vi "4Pi Obj Lock - Setup Camera.vi"(0 "Camera Notifier Name":string, 2 "Save ROI?":bool) -> (8 "Canceled?":bool)   [LabVIEW 2016]
uses:
  <vilib>/Utility/miscctls.llb/LVPointTypeDef.ctl
  Device Library/Cameras/Camera Controls/Generic Camera ROI.ctl
  Device Library/Cameras/Camera Controls/Generic Camera Actions.ctl
  4Pi Objective Lock Type Defs/4Pi Obj Lock - Camera Settings.ctl
panel:
  in  "Exposure Time (ms)":dbl
  in  "Tool Selection":enum32{"Zoom Tool", "ROI Tool", "Pan Tool"}(radio)
  in  "Cancel":bool
  in  "Done":bool
  out "Camera Display":T1(plugin-control)
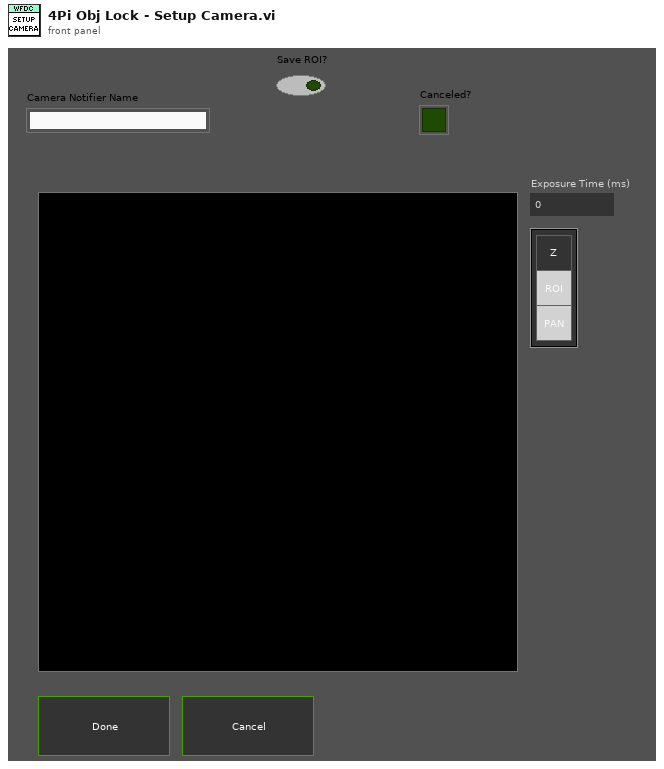
[diagram p1: front panel]
types:
  T1 = typedef "IMAQ Image.ctl" = refnum<image>
  T2 = typedef "Generic Camera Actions.ctl" = enum16{"Status", "Live Preview", "Capture", "Abort", "Set Exposure Time (s)", "Get Exposure Time (s)", "Record Settings", "Set ROI", "Get ROI", "Defect Correction On/Off", "Cooler On/Off", "Fan On/Off", "Quti"}
  T3 = typedef "Generic Camera ROI.ctl" = cluster{"H Offset":u16, "V Offset":u16, "H Width":u16, "V Width":u16}
  T4 = enum16{"Always On", "Always Off", "Off While Running"}
  T5 = typedef "LVPointTypeDef.ctl" = cluster{"Horizontal":i16, "Vertical":i16}
  T6 = typedef "LVRectTypeDef.ctl" = cluster{"Left":i16, "Top":i16, "Right":i16, "Bottom":i16}
  T7 = typedef "LVBoundsTypeDef.ctl" = cluster{"Width":u32, "Height":u32}
  T8 = typedef "4Pi Obj Lock - Camera Settings.ctl" = cluster{"Exposure Time (s)":dbl, "H Offset":u16, "V Offset":u16, "H Width":u16, "V Width":u16}
  T9 = cluster{"Global Rectangle":i32[], "Contours":cluster{"Contour Type":u32, "ROI Type":u32, "Points":i32[]}[]}
  T10 = cluster{"Contour Type":u32, "ROI Type":u32, "Points":i32[]}[]
  T11 = cluster{"Contour Type":u32, "ROI Type":u32, "Points":i32[]}
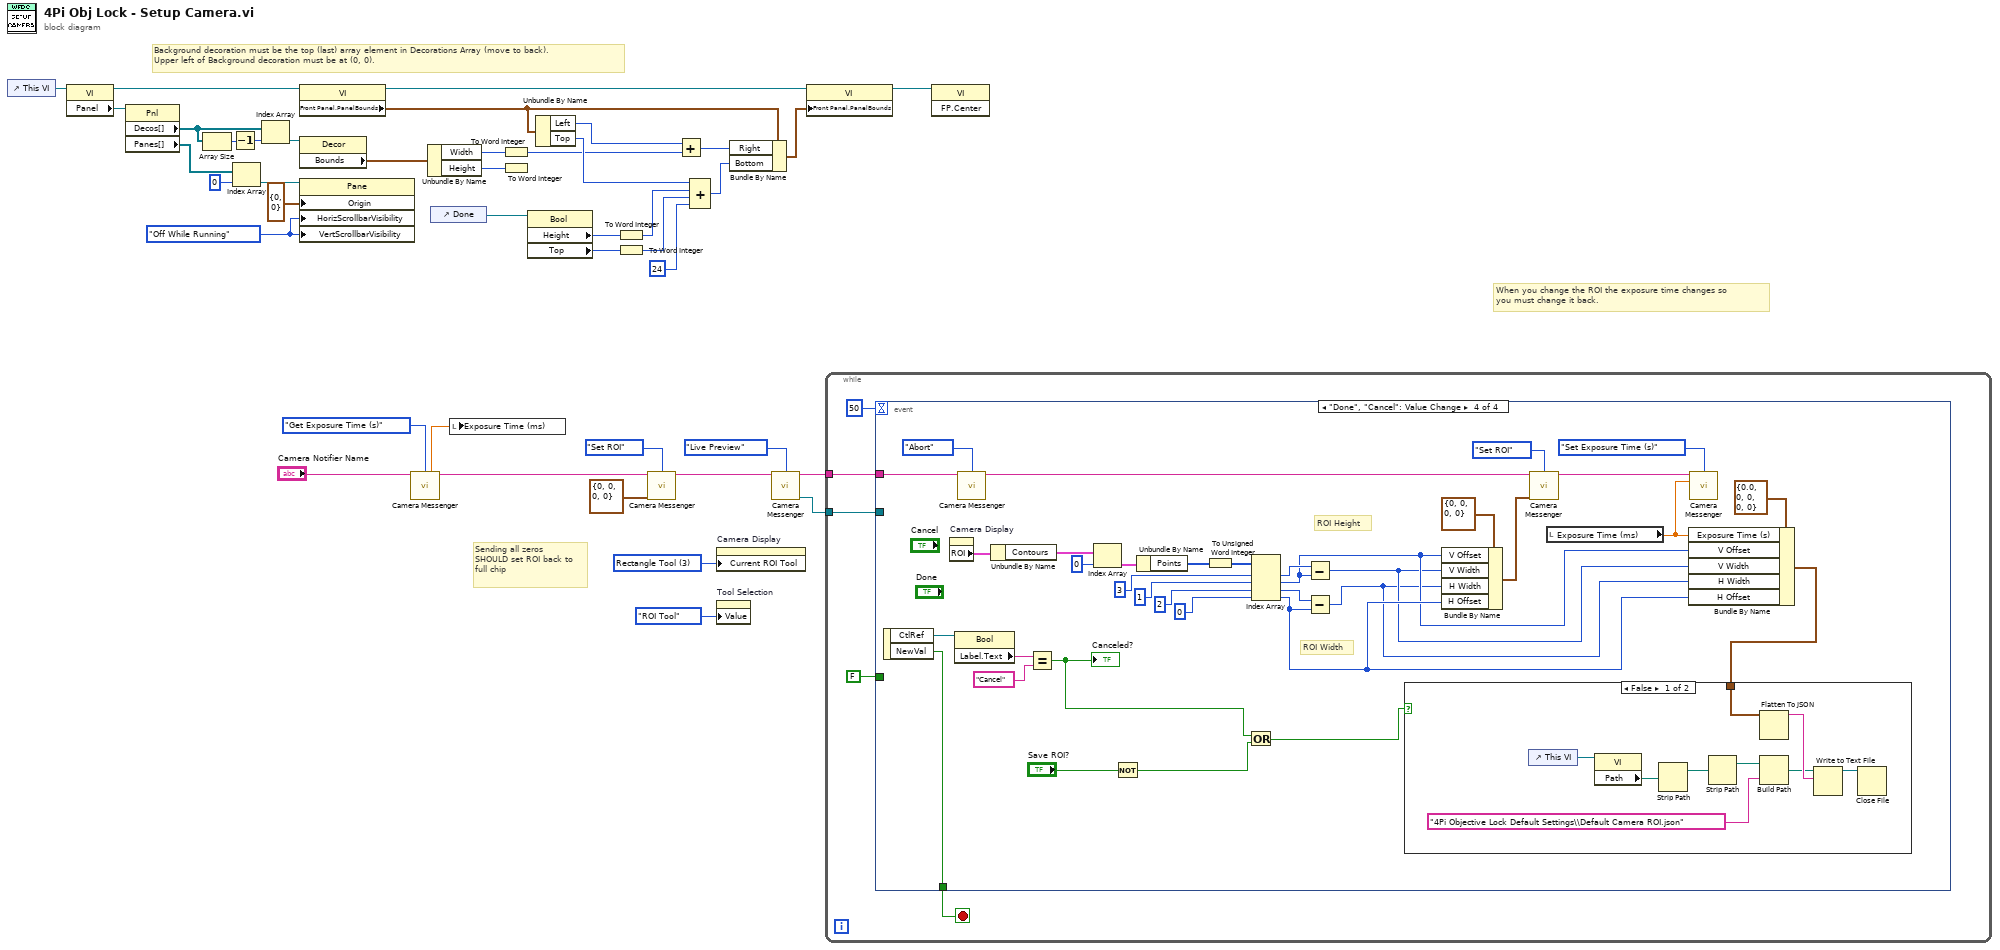
[diagram p0: block diagram]
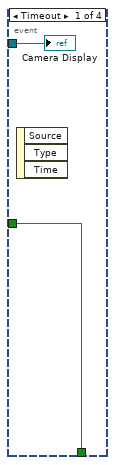
[diagram p2: hidden frame]
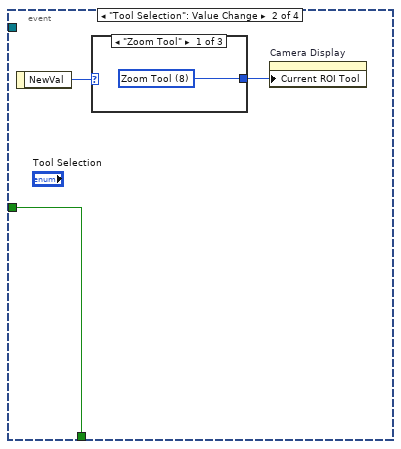
[diagram p3: hidden frame]
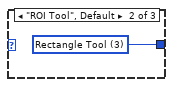
[diagram p4: hidden frame]
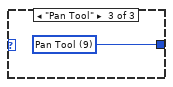
[diagram p5: hidden frame]
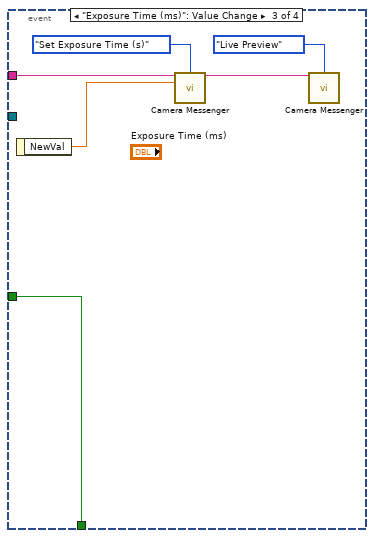
[diagram p6: hidden frame]
diagram:
  w23 = T4."Off While Running" ("Vertical Scrollbar Visibility")
  w42 = u32 3 items=["Zoom Tool"=8, "Selection Tool"=0, "Pan Tool"=9, "Point Tool"=1, "Line Tool"=2, "Rectangle Tool"=3, "Rotated Rectangle Tool"=12, "Polyline Tool"=10, "Polygon Tool"=5, "Freehand Tool"=11, "Closed Freehand Tool"=6, "Ellipse Tool"=4, "Annulus Tool"=7] ("Current ROI Tool")
  # "Background decoration must be the top (last) array element in Decorations Array (move to back).\nUpper left of Background decoration must be at (0, 0)."
  # "When you change the ROI the exposure time changes so\nyou must change it back."
  # "Sending all zeros SHOULD set ROI back to full chip"
  n1 = control-ref of="This VI"() -> (w15:refnum<vi>)
  n2 = property class="VI"(reference=w15) -> (reference out=w24:refnum<vi>, "Panel"=w16:refnum<vi>)  [unwired: 1 in, 1 out]
  n3 = property class="Pnl"(reference=w16) -> ("Decos[]"=w14:refnum<vi>[], "Panes[]"=w20:refnum<vi>[])  [unwired: 1 in, 2 out]
  n4 = Array Size(array=w14) -> (size(s)=w12:i32)
  n5 = Decrement(x=w12) -> (x-1=w13:i32)
  n6 = Index Array(array=w20, index=0) -> (element=w19:refnum<vi>)
  n7 = Index Array(array=w14, index=w13) -> (element=w22:refnum<vi>)
  n8 = property class="VI"(reference=w24) -> (reference out=w26:refnum<vi>, "Front Panel.PanelBounds"=w27:T6)  [unwired: 1 in, 1 out]
  n9 = property class="Decor"(reference=w22) -> ("Bounds"=w25:T7)  [unwired: 1 in, 2 out]
  n10 = property class="Pane"(reference=w19, "Origin"=T5 {"Horizontal"=0, "Vertical"=0}, "HorizScrollbarVisibility"=w23, "VertScrollbarVisibility"=w23) -> ()  [unwired: 1 in, 2 out]
  n11 = call "Camera Messenger.vi"("Notifier Name"="Camera Notifier Name", "General Camera Actions"=Generic_Camera_Actions."Get Exposure Time (s)") -> ("Current Exposure Time (s)"=w8:dbl, "Notifier Name Dup"=w7:string)  [unwired: 8 in, 4 out]
  n12 = Unbundle By Name(w25) -> ("Width"=w30:u32, "Height"=w33:u32)
  n13 = control-ref of="Done"() -> (w17:refnum<vi>)
  n14 = local write "Exposure Time (ms)"(w8) -> ()
  n15 = To Word Integer(number=w30) -> (16bit integer=w32:i16)
  n16 = To Word Integer(number=w33) -> ()  [unwired: 1 out]
  n17 = property class="Bool"(reference=w17) -> ("Height"=w35:u32, "Top"=w36:i32)  [unwired: 1 in, 2 out]
  n18 = Unbundle By Name(w27) -> ("Left"=w29:i16, "Top"=w40:i16)
  n19 = To Word Integer(number=w35) -> (16bit integer=w38:i16)
  n20 = To Word Integer(number=w36) -> (16bit integer=w39:i16)
  n21 = call "Camera Messenger.vi"("Notifier Name"=w7, "General Camera Actions"=Generic_Camera_Actions."Set ROI", "Camera ROI"=T3 {"H Offset"=0, "V Offset"=0, "H Width"=0, "V Width"=0} ("General Camera ROI")) -> ("Notifier Name Dup"=w4:string)  [unwired: 7 in, 5 out]
  n22 = Add(x=w29, y=w32) -> (x+y=w31:i16)
  n23 = Compound Arithmetic op=ADD(w40, w38, w39, i16 24 ("y")) -> (w34:i16)
  n24 = property on="Camera Display" class="ImageControl"("Current ROI Tool"=w42) -> ()  [unwired: 2 in, 2 out]
  n25 = property on="Tool Selection" class="RadioBtnsControl (strict)"("Value"=enum32{"Zoom Tool", "ROI Tool", "Pan Tool"}."ROI Tool" ("Tool Selection")) -> ()  [unwired: 2 in, 2 out]
  n26 = Bundle By Name(cluster=w27, "Right"=w31, "Bottom"=w34) -> (w28:T6)
  n27 = call "Camera Messenger.vi"("Notifier Name"=w4, "General Camera Actions"=Generic_Camera_Actions."Live Preview") -> ("Notifier Name Dup"=w3:string, "Image Ref"=w1:T1)  [unwired: 8 in, 4 out]
  n28 = property class="VI"(reference=w26, "Front Panel.PanelBounds"=w28) -> (reference out=w11:refnum<vi>)  [unwired: 1 in, 1 out]
  n29 = while {
    tunnel: w1 -> [w45]
    tunnel: w3 -> [w43]
    stop <- w47 stop-if-true
    n30 = event shown="[3] \"Done\", \"Cancel\": Value Change" {
      selector: _ -> [_ _ _ _]
      dyn-events: _ -> [_ _ _ _]
      timeout: 50 -> [_ _ _ _]
      tunnel: [w49 w52 w61 w93] -> w47
      tunnel: FALSE -> [w49 w52 w61 _]
      tunnel: w45 -> [w48 _ _ _]
      tunnel: w43 -> [_ _ w60 w81]
      event Timeout {
        n31 = event-data() -> ()  [unwired: 1 in, 3 out]
        "Camera Display" <- w48
      }
      event "Tool Selection": Value Change {
        n32 = event-data() -> ("NewVal"=w51:enum32{"Zoom Tool", "ROI Tool", "Pan Tool"})  [unwired: 1 in]
        n33 = case shown="\"Zoom Tool\"" w51 {
          tunnel: [w53 w54 w55] -> w50
          frame "Zoom Tool" {
            w53 = u32 8 items=["Zoom Tool"=8, "Selection Tool"=0, "Pan Tool"=9, "Point Tool"=1, "Line Tool"=2, "Rectangle Tool"=3, "Rotated Rectangle Tool"=12, "Polyline Tool"=10, "Polygon Tool"=5, "Freehand Tool"=11, "Closed Freehand Tool"=6, "Ellipse Tool"=4, "Annulus Tool"=7] ("Current ROI Tool")
          }
          frame "ROI Tool", Default {
            w54 = u32 3 items=["Zoom Tool"=8, "Selection Tool"=0, "Pan Tool"=9, "Point Tool"=1, "Line Tool"=2, "Rectangle Tool"=3, "Rotated Rectangle Tool"=12, "Polyline Tool"=10, "Polygon Tool"=5, "Freehand Tool"=11, "Closed Freehand Tool"=6, "Ellipse Tool"=4, "Annulus Tool"=7] ("Current ROI Tool")
          }
          frame "Pan Tool" {
            w55 = u32 9 items=["Zoom Tool"=8, "Selection Tool"=0, "Pan Tool"=9, "Point Tool"=1, "Line Tool"=2, "Rectangle Tool"=3, "Rotated Rectangle Tool"=12, "Polyline Tool"=10, "Polygon Tool"=5, "Freehand Tool"=11, "Closed Freehand Tool"=6, "Ellipse Tool"=4, "Annulus Tool"=7] ("Current ROI Tool")
          }
        }
        n34 = property on="Camera Display" class="ImageControl"("Current ROI Tool"=w50) -> ()  [unwired: 2 in, 2 out]
      }
      event "Exposure Time (ms)": Value Change {
        n35 = event-data() -> ("NewVal"=w58:dbl)  [unwired: 1 in]
        n36 = call "Camera Messenger.vi"("Notifier Name"=w60, "General Camera Actions"=Generic_Camera_Actions."Set Exposure Time (s)", "Exposure Time (s)"=w58) -> ("Notifier Name Dup"=w57:string)  [unwired: 7 in, 5 out]
        n37 = call "Camera Messenger.vi"("Notifier Name"=w57, "General Camera Actions"=Generic_Camera_Actions."Live Preview") -> ()  [unwired: 8 in, 6 out]
      }
      event "Done", "Cancel": Value Change {
        # "ROI Width"
        # "ROI Height"
        n38 = event-data() -> ("CtlRef"=w96:refnum<vi>, "NewVal"=w93:bool)  [unwired: 1 in]
        n39 = property on="Camera Display" class="ImageControl"() -> ("ROI"=w89:T9)  [unwired: 2 in, 2 out]
        n40 = property class="Bool"(reference=w96) -> ("Label.Text"=w95:string)  [unwired: 1 in, 2 out]
        n41 = call "Camera Messenger.vi"("Notifier Name"=w81, "General Camera Actions"=Generic_Camera_Actions."Abort") -> ("Notifier Name Dup"=w78:string)  [unwired: 8 in, 5 out]
        n42 = Unbundle By Name(w89) -> ("Contours"=w88:T10)
        n43 = Equal?(x=w95, y="Cancel") -> (x = y?=w64:bool)
        "Canceled?" <- w64
        n44 = Index Array(array=w88, index=0) -> (element=w87:T11)
        n45 = Not(x="Save ROI?") -> (.not. x?=w63:bool)
        n46 = Unbundle By Name(w87) -> ("Points"=w90:i32[])
        n47 = To Unsigned Word Integer(number=w90) -> (unsigned 16bit integer=w71:u16[])
        n48 = Or(x=w64, y=w63) -> (x .or. y?=w62:bool)
        n49 = Index Array(array=w71, index #1=3 ("index"), index #2=1 ("index"), index #3=2 ("index"), index #4=0 ("index")) -> (element #1=w92:u16, element #2=w69:u16, element #3=w91:u16, element #4=w70:u16)
        n50 = Subtract(x=w92, y=w69) -> (x-y=w68:u16)
        n51 = Subtract(x=w91, y=w70) -> (x-y=w67:u16)
        n52 = Bundle By Name(cluster=T3 {"H Offset"=0, "V Offset"=0, "H Width"=0, "V Width"=0} ("General Camera ROI"), "V Offset"=w69, "V Width"=w68, "H Width"=w67, "H Offset"=w70) -> (w77:T3)
        n53 = call "Camera Messenger.vi"("Notifier Name"=w78, "General Camera Actions"=Generic_Camera_Actions."Set ROI", "Camera ROI"=w77) -> ("Notifier Name Dup"=w75:string)  [unwired: 7 in, 5 out]
        n54 = local read "Exposure Time (ms)"() -> (w72:dbl)
        n55 = Bundle By Name(cluster=T8 {"Exposure Time (s)"=0.0, "H Offset"=0, "V Offset"=0, "H Width"=0, "V Width"=0} ("Camera Settings"), "Exposure Time (s)"=w72, "V Offset"=w69, "V Width"=w68, "H Width"=w67, "H Offset"=w70) -> (w66:T8)
        n56 = case shown="False" w62 {
          tunnel: w66 -> [w97 _]
          frame False {
            n57 = control-ref of="This VI"() -> (w100:refnum<vi>)
            n58 = property class="VI"(reference=w100) -> ("Path"=w99:path)  [unwired: 1 in, 2 out]
            n59 = Strip Path(path=w99) -> (stripped path=w101:path)  [unwired: 1 out]
            n60 = Strip Path(path=w101) -> (stripped path=w102:path)  [unwired: 1 out]
            n61 = Flatten To JSON(anything=w97) -> (JSON string=w104:string)  [unwired: 2 in, 1 out]
            n62 = Build Path(base path=w102, name or relative path="4Pi Objective Lock Default Settings\\Default Camera ROI.json") -> (appended path=w98:path)
            n63 = Write to Text File(file (use dialog)=w98, text=w104) -> (refnum out=w105:refnum<file>)  [unwired: 2 in, 2 out]
            n64 = Close File(refnum=w105) -> ()  [unwired: 1 in, 2 out]
          }
          frame True {
          }
        }
        n65 = call "Camera Messenger.vi"("Notifier Name"=w75, "General Camera Actions"=Generic_Camera_Actions."Set Exposure Time (s)", "Exposure Time (s)"=w72) -> ()  [unwired: 7 in, 6 out]
      }
    }
  }
  n66 = invoke class="VI" method="FP.Center"(reference=w11) -> ()  [unwired: 2 in, 3 out]
